vi "Get Tree Indentation Levels.vi"(8 "error in (no error)":errorcluster, 11 "Message Array":refnum<class "Message.lvclass">[](array[class])) -> (0 "error out":errorcluster, 2 "Tree indentation level Array":i32[](array[numeric]), 3 "Class Base Name Array":string[](array[string]))   [LabVIEW 2020, in "Sequencer.lvlib"]
doc: "Get Class Base Names and indentation levels from the 'Message Array'."
uses:
  Sequencer.lvlib
  PPL/HDH.Actor Framework.Core.Actor.lvlibp/1abvi3w/vi.lib/ActorFramework/Message/Message.lvclass
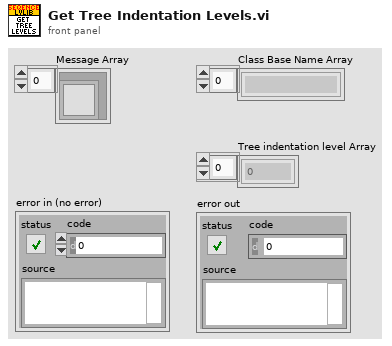
[diagram p1: front panel]
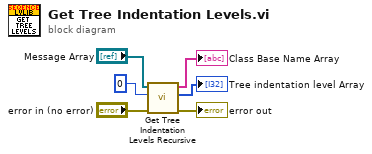
[diagram p0: block diagram]
diagram:
  n1 = call "Get Tree Indentation Levels Recursive.vi"("error in (no error)"="error in (no error)", "Initial tree level"=0, "Message Array"="Message Array") -> ("error out"=→"error out":errorcluster, "Tree indentation level Array"=→"Tree indentation level Array":i32[], "Class Base Name Array"=→"Class Base Name Array":string[])  [unwired: 6 in]
